vi "Iterator_Create.vi"(0 "reference in":refnum<class "Iterator.lvclass">, 5 "error in (no error)":errorcluster) -> (14 "reference out":refnum<class "Iterator.lvclass">, 19 "error out":errorcluster)   [LabVIEW 2015, in "Iterator.lvclass"]
uses:
  Iterator.lvclass
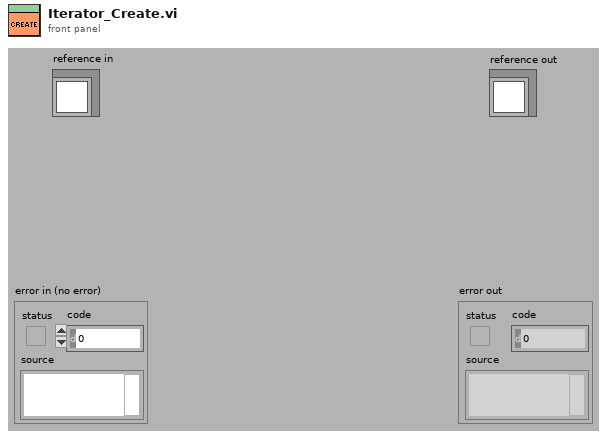
[diagram p1: front panel]
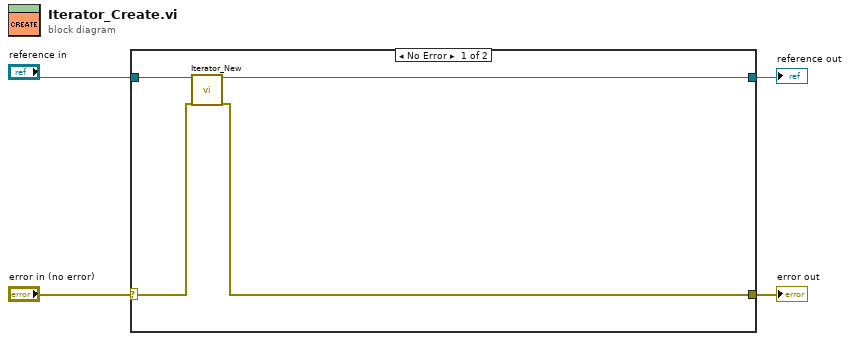
[diagram p0: block diagram]
diagram:
  n1 = case shown="No Error" "error in (no error)" {
    selector: "error in (no error)" -> [w6 w10]
    tunnel: [w5 w10] -> w3
    tunnel: "reference in" -> [w8 w9]
    tunnel: [w7 w9] -> w1
    frame No Error {
      n2 = call "Iterator_New.vi"("reference in"=w8, "error in (no error)"=w6) -> ("reference out"=w7:refnum<class "Iterator.lvclass">, "error out"=w5:errorcluster)  [unwired: 14 in, 2 out]
    }
    frame Error {
    }
  }
  "error out" <- w3
  "reference out" <- w1
